vi "MeteoStation.vi"() -> ()   [LabVIEW 2020]
uses:
  <vilib>/Instr/_visa.llb/VISA Configure Serial Port (Instr).vi
panel:
  out "LED 3":bool
  out "LED 2":bool
  in  "Chart size, hours":dbl(slide) step=0.25 scale=0.25..54.0
  out "LED 1":bool
  out "Status":string
  out "LogFile at...":path
  out "Start time":string
  out "Light":string
  out "Altitude":string
  out "Pressure":string
  out "Temp DH21":string
  out "Number of measurements":dbl
  out "Time of the last sensor survey":string
  in  "Stop Button":bool
  in  "Resource name":refnum<visa-resource-name>="COM7"
  out "Temp DS18B20":string
  out "Humidity":string
  out "Temp BMP180":string
  out "Air humidity graph":waveform(dbl)(graph)
  out "Temperature graph":waveform(dbl)[](graph)
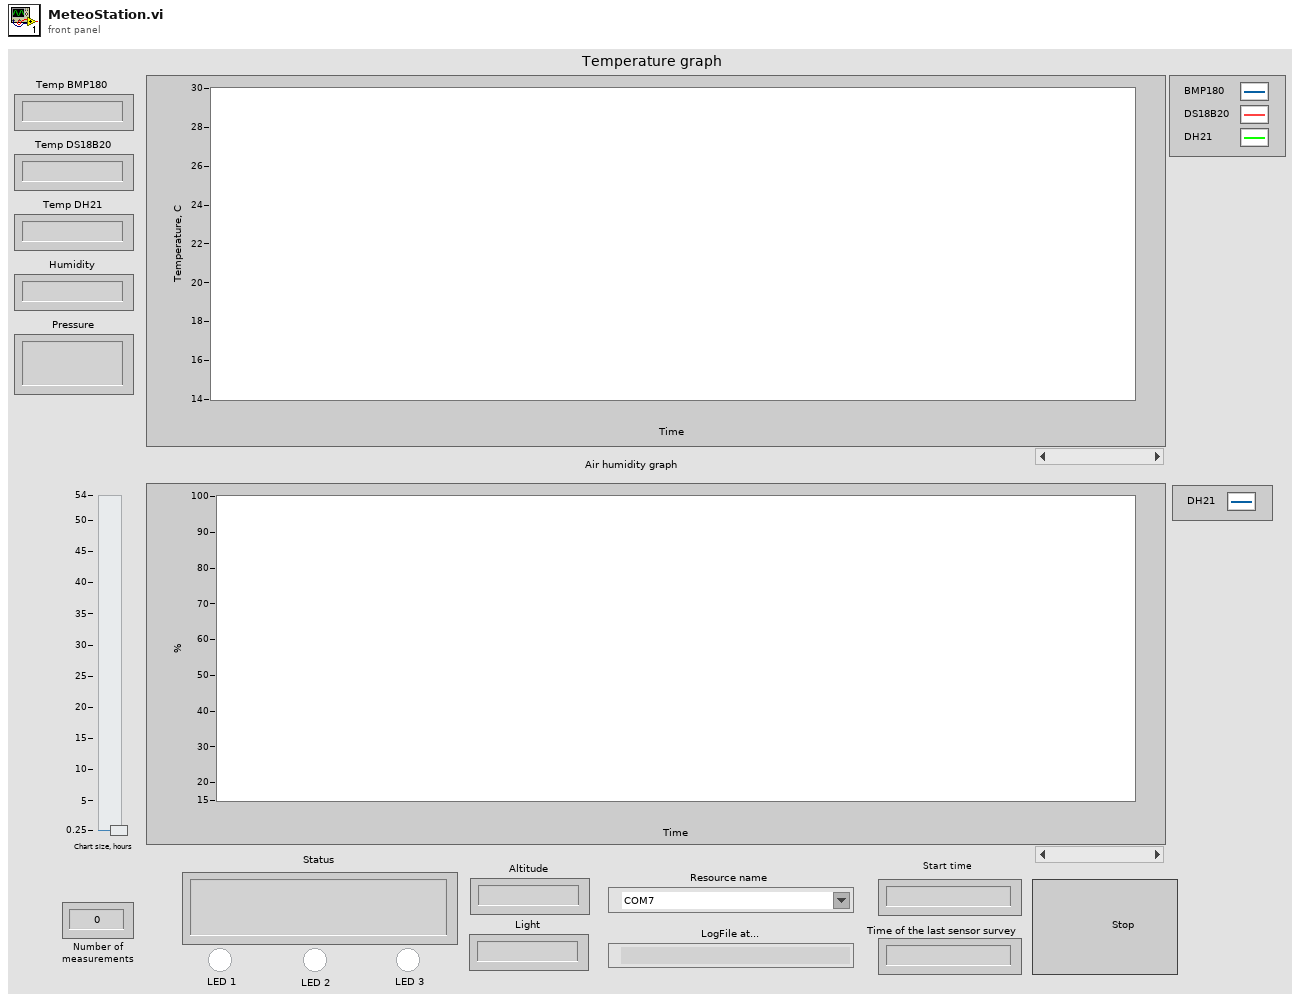
[diagram p1: front panel]
types:
  T1 = enum16{"open", "replace", "create", "open or create", "replace or create", "replace or create with confirmation"}
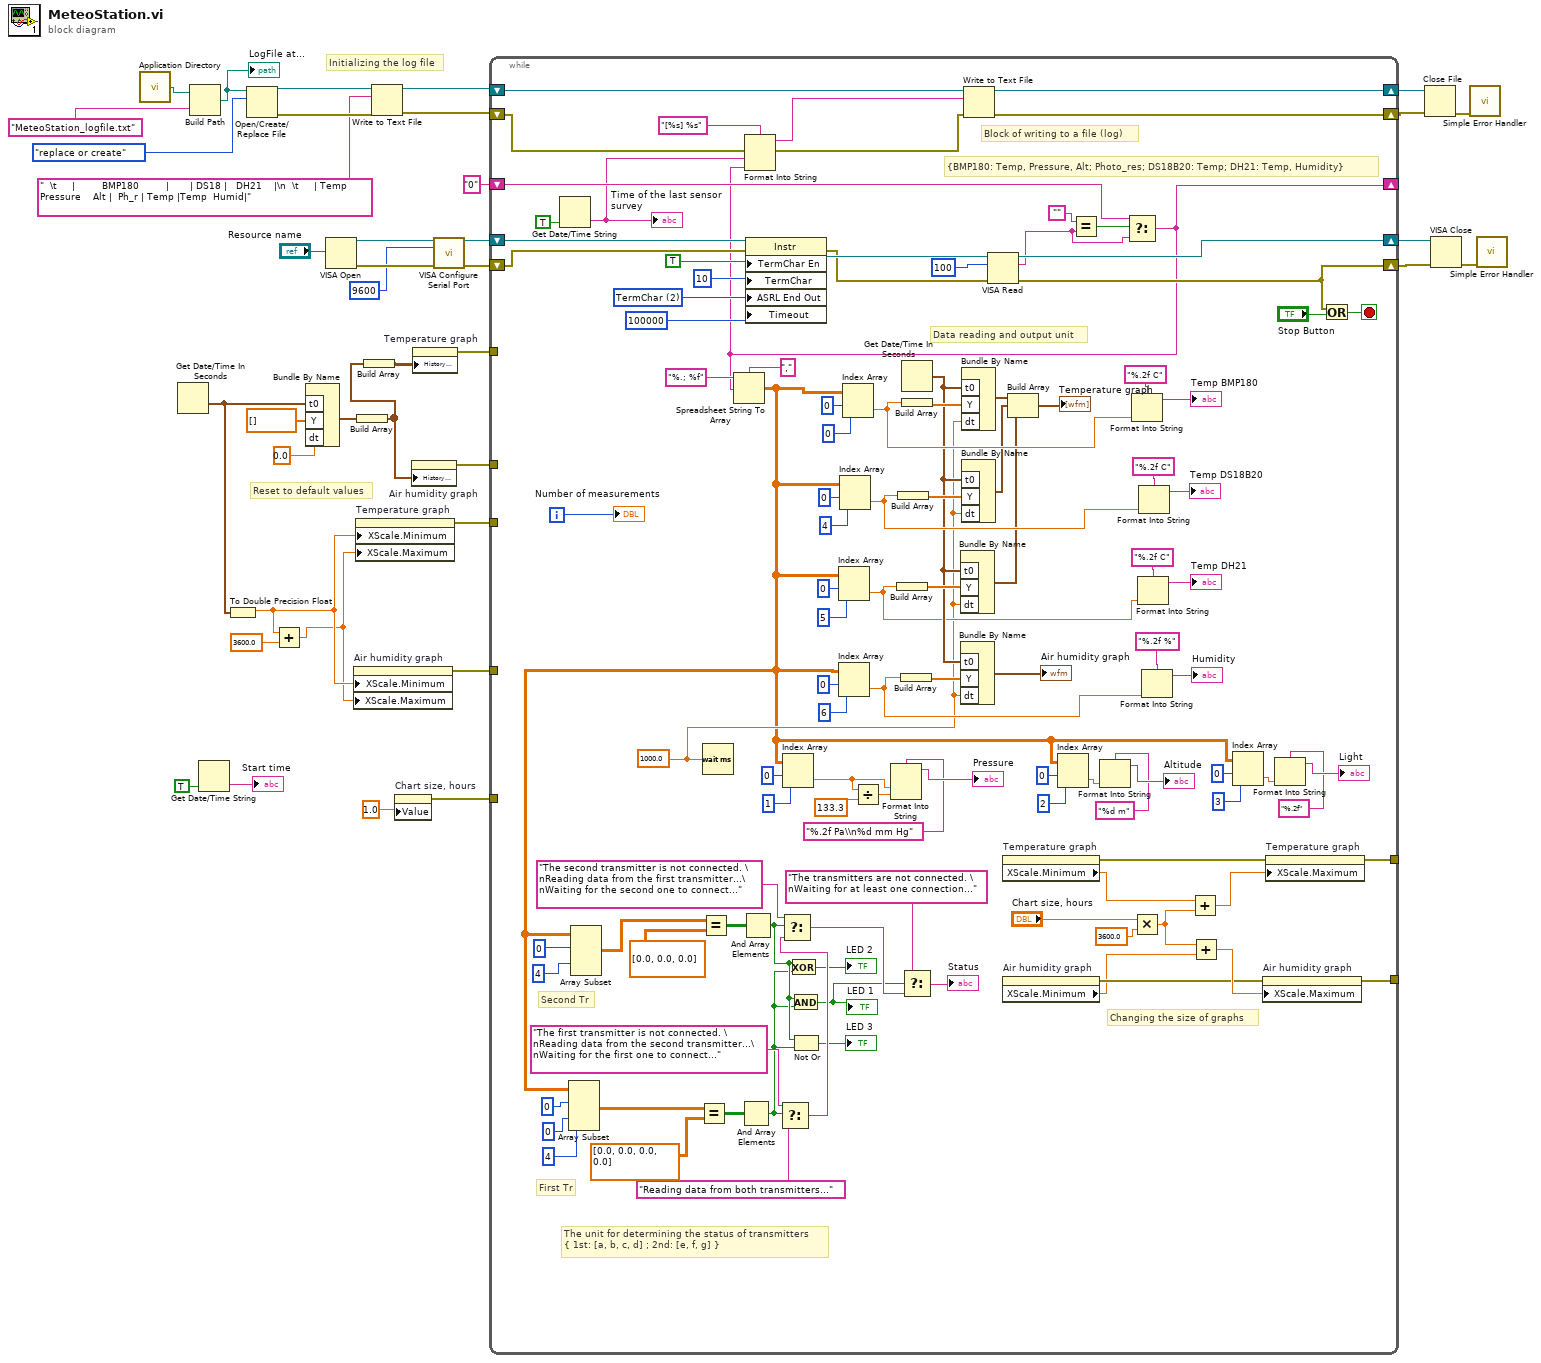
[diagram p0: block diagram]
diagram:
  # "Initializing the log file"
  # "Reset to default values"
  n1 = call <vilib>:"Application Directory.vi"() -> ("Application Directory"=w21:path)
  n2 = Get Date/Time In Seconds() -> (seconds since 1Jan1904=w28:timestamp)
  n3 = Build Path(base path=w21, name or relative path="MeteoStation_logfile.txt") -> (appended path=w17:path)
  "LogFile at..." <- w17
  n4 = Get Date/Time String(want seconds? (F)=TRUE) -> (time string=→"Start time":string)  [unwired: 2 in, 1 out]
  n5 = To Double Precision Float(number=w28) -> (double precision float=w30:dbl)
  n6 = Open/Create/Replace File(file path (use dialog)=w17, operation (0:open)=T1."replace or create") -> (refnum out=w7:refnum<file>, error out=w6:errorcluster)  [unwired: 4 in, 1 out]
  n7 = Add(x=w30, y=3600.0) -> (x+y=w29:dbl)
  n8 = Bundle By Name("t0"=w28, "Y"=dbl[] [], "dt"=0.0) -> (w24:waveform(dbl))  [unwired: 1 in]
  n9 = VISA Open(VISA resource name="Resource name") -> (VISA resource name=w14:refnum<visa-resource-name>, error out=w13:errorcluster)  [unwired: 4 in]
  n10 = property on="Air humidity graph" class="WFChart (strict)"("XScale.Minimum"=w30, "XScale.Maximum"=w29) -> (error out=w25:errorcluster)  [unwired: 2 in, 1 out]
  n11 = property on="Temperature graph" class="WFChart (strict)"("XScale.Minimum"=w30, "XScale.Maximum"=w29) -> (error out=w26:errorcluster)  [unwired: 2 in, 1 out]
  n12 = Build Array(w24) -> (w23:waveform(dbl)[])
  n13 = Build Array(w23) -> (w22:waveform(dbl)[][])
  n14 = Write to Text File(file (use dialog)=w7, text="  \t     |         BMP180         |       | DS18 |   DH21    |\n  \t     | Temp   Pressure    Alt |  Ph_r | Temp |Temp  Humid|" ("initial string"), error in=w6) -> (refnum out=w4:refnum<file>, error out=w5:errorcluster)  [unwired: 1 in, 1 out]
  n15 = property on="Chart size, hours" class="Slide (strict)"("Value"=1.0 ("Chart size, \nhours")) -> (error out=w1:errorcluster)  [unwired: 2 in, 1 out]
  n16 = property on="Air humidity graph" class="WFChart (strict)"("History Data"=w23) -> (error out=w36:errorcluster)  [unwired: 2 in, 1 out]
  n17 = property on="Temperature graph" class="WFChart (strict)"("History Data"=w22) -> (error out=w35:errorcluster)  [unwired: 2 in, 1 out]
  n18 = call-poly "VISA Configure Serial Port"("VISA resource name"=w14, "baud rate (9600)"=u32 9600 ("Serial Settings:Baud Rate"), "error in (no error)"=w13) -> ("VISA resource name out"=w12:refnum<visa-resource-name>, "error out"=w11:errorcluster)  [unwired: 11 in]
  n19 = while {
    shift-right: [w152] -> w39
    shift-left: w12 -> [w83]
    shift-right: [w150] -> w38
    shift-left: w11 -> [w82]
    shift-right: [w66] -> _
    shift-left: "0" ("read buffer") -> [w147]
    tunnel: w36 -> [_]
    tunnel: w35 -> [_]
    tunnel: w26 -> [_]
    tunnel: w25 -> [_]
    tunnel: [w120] -> _
    tunnel: [w119] -> _
    shift-right: [w72] -> w9
    shift-left: w4 -> [w73]
    shift-right: [w71] -> w8
    shift-left: w5 -> [w68]
    tunnel: w1 -> [_]
    i -> [w125]
    stop <- w151 stop-if-true
    w77 = u16 2 items=["None", "Last Bit", "TermChar", "Break"] ("Serial Settings:End Mode for Writes")
    w74 = 1000.0 ("y")
    # "Changing the size of graphs"
    # "The unit for determining the status of transmitters\n{ 1st: [a, b, c, d] ; 2nd: [e, f, g] }"
    # "Data reading and output unit"
    # "Block of writing to a file (log)"
    # "First Tr"
    # "Second Tr"
    # "{BMP180: Temp, Pressure, Alt; Photo_res; DS18B20: Temp; DH21: Temp, Humidity}"
    n20 = Get Date/Time String(want seconds? (F)=TRUE) -> (time string=w65:string)  [unwired: 2 in, 1 out]
    "Time of the last sensor survey" <- w65
    n21 = Wait (ms)(milliseconds to wait=w74) -> ()  [unwired: 1 out]
    n22 = property class="Instr"(reference=w83, error in=w82, "TermChar En"=TRUE ("Message Based Settings:Termination Character Enable"), "TermChar"=u32 10 ("Serial Settings:Baud Rate"), "ASRL End Out"=w77, "Timeout"=u32 100000 ("General Settings:Timeout Value")) -> (reference out=w81:refnum<visa-resource-name>, error out=w80:errorcluster)
    n23 = Get Date/Time In Seconds() -> (seconds since 1Jan1904=w104:timestamp)
    n24 = VISA Read(VISA resource name=w81, byte count=u32 100, error in (no error)=w80) -> (VISA resource name out=w152:refnum<visa-resource-name>, read buffer=w84:string, error out=w150:errorcluster)  [unwired: 1 out]
    n25 = property on="Temperature graph" class="WFChart (strict)"() -> (error out=w116:errorcluster, "XScale.Minimum"=w118:dbl)  [unwired: 2 in, 1 out]
    n26 = property on="Air humidity graph" class="WFChart (strict)"() -> (error out=w114:errorcluster, "XScale.Minimum"=w112:dbl)  [unwired: 2 in, 1 out]
    n27 = Equal?(x="", y=w84) -> (x = y?=w148:bool)
    n28 = Select(t=w147, s=w148, f=w84) -> (s? t:f=w66:string)
    n29 = Spreadsheet String To Array(delimiter (Tab)=",", format string="%.; %f", spreadsheet string=w66) -> (array=w63:dbl[][])  [unwired: 1 in]
    n30 = Array Subset(array=w63, index (row)=0 ("index"), index (col)=0 ("index"), length (col)=4 ("length")) -> (w53:dbl[][])  [unwired: 1 in]
    n31 = Array Subset(array=w63, index (row)=0 ("index"), index (col)=4 ("index")) -> (w58:dbl[][])  [unwired: 2 in]
    n32 = Equal?(x=w53, y=dbl[][] [[0.0, 0.0, 0.0, 0.0]]) -> (x = y?=w54:bool[][])
    n33 = Equal?(x=w58, y=dbl[][] [[0.0, 0.0, 0.0]]) -> (x = y?=w56:bool[][])
    n34 = And Array Elements(Boolean array=w54) -> (logical AND=w40:bool)
    n35 = And Array Elements(Boolean array=w56) -> (logical AND=w41:bool)
    n36 = Format Into String(format string="[%s] %s", error in=w68, w65, w66) -> (resulting string=w69:string, error out=w67:errorcluster)  [unwired: 1 in]
    n37 = Select(t="The first transmitter is not connected. \nReading data from the second transmitter...\nWaiting for the first one to connect...", s=w40, f="Reading data from both transmitters...") -> (s? t:f=w50:string)
    n38 = Select(t="The second transmitter is not connected. \nReading data from the first transmitter...\nWaiting for the second one to connect...", s=w41, f=w50) -> (s? t:f=w45:string)
    n39 = Index Array(array=w63, index (row)=0, index (col)=1 ("disabled index (col)")) -> (element=w86:dbl)
    n40 = Exclusive Or(1:w40, 2:w41) -> (0:→"LED 2":bool)
    n41 = And(x=w41, y=w40) -> (x .and. y?=w43:bool)
    "LED 1" <- w43
    n42 = Not Or(1:w40, 2:w41) -> (0:→"LED 3":bool)
    n43 = Index Array(array=w63, index (row)=0, index (col)=5 ("disabled index (col)")) -> (element=w102:dbl)
    n44 = Index Array(array=w63, index (row)=0, index (col)=6 ("disabled index (col)")) -> (element=w110:dbl)
    n45 = Index Array(array=w63, index (row)=0, index (col)=4 ("disabled index (col)")) -> (element=w111:dbl)
    n46 = Index Array "Index Array"(array=w63, index (row)=0, index (col)=0 ("disabled index (col)")) -> (element=w126:dbl)
    n47 = Divide(x=w86, y=133.3) -> (x/y=w87:dbl)
    n48 = Format Into String(format string="%.2f Pa\\n%d mm Hg", w86, w87) -> (resulting string=→"Pressure":string)  [unwired: 2 in, 1 out]
    n49 = Build Array(w102) -> (w105:dbl[])
    n50 = Build Array(w111) -> (w128:dbl[])
    n51 = Build Array(w110) -> (w127:dbl[])
    n52 = Build Array(w126) -> (w129:dbl[])
    n53 = Select(t="The transmitters are not connected. \nWaiting for at least one connection...", s=w43, f=w45) -> (s? t:f=→"Status":string)
    n54 = Bundle By Name("t0"=w104, "Y"=w105, "dt"=w74) -> (w103:waveform(dbl))  [unwired: 1 in]
    n55 = Bundle By Name("t0"=w104, "Y"=w127, "dt"=w74) -> (→"Air humidity graph":waveform(dbl))  [unwired: 1 in]
    n56 = Bundle By Name("t0"=w104, "Y"=w129, "dt"=w74) -> (w124:waveform(dbl))  [unwired: 1 in]
    n57 = Bundle By Name("t0"=w104, "Y"=w128, "dt"=w74) -> (w123:waveform(dbl))  [unwired: 1 in]
    n58 = Write to Text File(file (use dialog)=w73, text=w69, error in=w67) -> (refnum out=w72:refnum<file>, error out=w71:errorcluster)  [unwired: 1 in, 1 out]
    n59 = Build Array(w124, w123, w103) -> (→"Temperature graph":waveform(dbl)[])
    n60 = Index Array(array=w63, index (row)=0, index (col)=2 ("disabled index (col)")) -> (element=w95:dbl)
    n61 = Format Into String(format string="%d m", w95) -> (resulting string=→"Altitude":string)  [unwired: 2 in, 1 out]
    n62 = Format Into String(format string="%.2f C", w126) -> (resulting string=→"Temp BMP180":string)  [unwired: 2 in, 1 out]
    n63 = Multiply(x="Chart size, hours", y=3600.0) -> (x*y=w113:dbl)
    n64 = Format Into String(format string="%.2f C", w102) -> (resulting string=→"Temp DH21":string)  [unwired: 2 in, 1 out]
    n65 = Format Into String(format string="%.2f C", w111) -> (resulting string=→"Temp DS18B20":string)  [unwired: 2 in, 1 out]
    n66 = Format Into String(format string="%.2f %", w110) -> (resulting string=→"Humidity":string)  [unwired: 2 in, 1 out]
    n67 = Add(x=w118, y=w113) -> (x+y=w117:dbl)
    n68 = Add(x=w113, y=w112) -> (x+y=w115:dbl)
    n69 = Index Array(array=w63, index (row)=0, index (col)=3 ("disabled index (col)")) -> (element=w92:dbl)
    n70 = property on="Air humidity graph" class="WFChart (strict)"(error in=w114, "XScale.Maximum"=w115) -> (error out=w119:errorcluster)  [unwired: 1 in, 1 out]
    n71 = property on="Temperature graph" class="WFChart (strict)"(error in=w116, "XScale.Maximum"=w117) -> (error out=w120:errorcluster)  [unwired: 1 in, 1 out]
    n72 = Format Into String(format string="%.2f", w92) -> (resulting string=→"Light":string)  [unwired: 2 in, 1 out]
    n73 = Or(x=w150, y="Stop Button") -> (x .or. y?=w151:bool)
    "Number of measurements" <- w125
  }
  n74 = Close File(refnum=w9, error in=w8) -> (error out=w15:errorcluster)  [unwired: 1 out]
  n75 = VISA Close(VISA resource name=w39, error in (no error)=w38) -> (error out=w37:errorcluster)
  n76 = call <vilib>:"Simple Error Handler.vi"("error in (no error)"=w15) -> ()  [unwired: 4 in, 5 out]
  n77 = call <vilib>:"Simple Error Handler.vi"("error in (no error)"=w37) -> ()  [unwired: 4 in, 5 out]
